vi "System Name.vi"(11 "VolatusAPI in":refnum<class "VolatusAPI.lvclass">) -> (2 "System":string, 3 "VolatusAPI out":refnum<class "VolatusAPI.lvclass">)   [LabVIEW 2020, in "Volatus.lvlib" / "VolatusAPI.lvclass"]
uses:
  VolatusAPI.lvclass
  VolatusAPI.lvclass/VolatusAPI.ctl
  lv-vecto/Vecto/Vecto/Vecto.lvclass
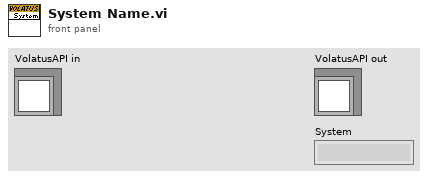
[diagram p1: front panel]
types:
  T1 = typedef "VectoConfig.lvlib/Node Info.ctl" = cluster{"System":string, "Cluster":string, "Name":string, "ID":u32, "Capabilities":string[]}
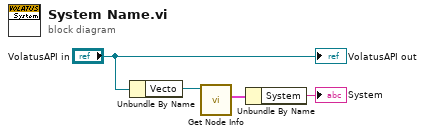
[diagram p0: block diagram]
diagram:
  n1 = Unbundle By Name("VolatusAPI in") -> ("Vecto"=w3:refnum<class "Vecto.lvclass">)
  n2 = call "Get Node Info.vi"("Vecto in"=w3) -> ("Info"=w2:T1)  [unwired: 8 in, 2 out]
  n3 = Unbundle By Name(w2) -> ("System"=→"System":string)
  "VolatusAPI out" <- "VolatusAPI in"
